vi "Frame to ROI Frame.vi"(1 "Apply? (T)":bool=TRUE, 2 "ROI Descriptor":T1 {"Contours"."Type" items=["No Selection", "Point", "Line", "Rectangle", "Oval", "Polygon", "Freehand Region", "Annulus", "Unused2", "Unused3", "Broken Line", "Freehand Line", "Rotated Rectangle"]}, 3 "Video Frame":refnum<class "Video Frame.lvclass">) -> (0 "ROIed Video Frame":refnum<class "ROIed Video Frame.lvclass">)   [LabVIEW 2018]
uses:
  Classes/Video Frame/Video Frame.lvclass
  Classes/ROIed Video Frame/ROIed Video Frame.lvclass
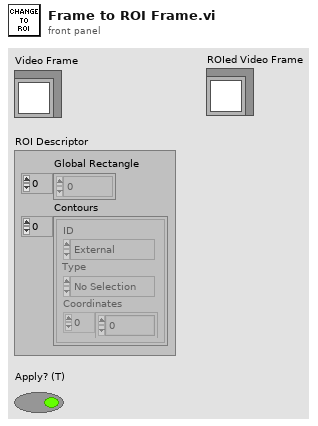
[diagram p1: front panel]
types:
  T1 = typedef "ROI Descriptor" = cluster{"Global Rectangle":i32[], "Contours":cluster{"ID":enum32{"External", "Internal"}, "Type":u32, "Coordinates":i32[]}[]}
  T2 = typedef "IMAQ Image.ctl" = refnum<image>
  T3 = cluster{"Width":u32, "Height":u32, "Frames Per Second":u32, "Codec":string, "Has Data":bool}
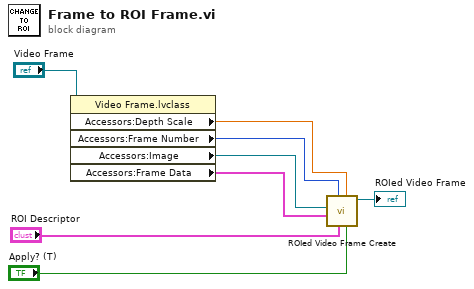
[diagram p0: block diagram]
diagram:
  n1 = property class="Video Frame.lvclass"(reference="Video Frame") -> ("Accessors:Depth Scale"=w7:dbl, "Accessors:Frame Number"=w6:i32, "Accessors:Image"=w5:T2, "Accessors:Frame Data"=w4:T3)  [unwired: 1 in, 2 out]
  n2 = call "ROIed Video Frame Create.vi"("Apply? (T)"="Apply? (T)", "Depth Scale"=w7, "ROI Descriptor"="ROI Descriptor", "Frame Number"=w6, "Frame Data"=w4, "Image Dst"=w5) -> ("ROIed Video Frame out"=→"ROIed Video Frame":refnum<class "ROIed Video Frame.lvclass">)  [unwired: 4 in, 1 out]
